vi "TEST LVOOP Plug Ins - Cluster.vi"() -> (0 "Cluster":T1)   [LabVIEW 2009]
doc: "This is the Cluster VI for the test stub VI for the LVOOP Plug Ins Exercise.\n\nAAL 9/09"
uses:
  Report Class/Report.lvclass
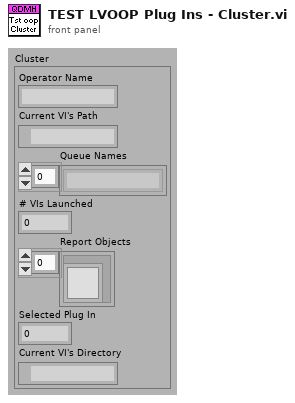
[diagram p1: front panel]
types:
  T1 = cluster{"Operator Name":string, "Current VI's Path":path, "Queue Names":string[], "# VIs Launched":i32, "Report Objects":refnum<class "Report.lvclass">[], "Selected Plug In":i32, "Current VI's Directory":path}
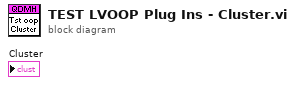
[diagram p0: block diagram]
diagram:
